vi "BELIKIN FPGA Interface.vi"() -> ()   [LabVIEW 2015]
uses:
  IP Dev Area/IP results.ctl
  <vilib>/Utility/miscctls.llb/LVRectTypeDef.ctl
  <vilib>/userdefined/High Color/IMAQdx.ctl
  <vilib>/FPGAPlugInAG/cRIO-9030/niLvFpga_Open_cRIO-9030.vi
  <vilib>/rvi/interface/common/dynamic/niFpgaDynamicAddResources.vi
  <vilib>/FPGAPlugInAG/Dynamic/niLvFpga_Download_Dynamic.vi
  <vilib>/FPGAPlugInAG/Dynamic/niLvFpga_Run_Dynamic.vi
  <vilib>/Utility/error.llb/Error Cluster From Error Code.vi
  <vilib>/rvi/errors/niLvFpgaAdjustHostInterfaceError.vi
  <vilib>/rvi/interface/nirviOpenFPGA/nirviOpenFPGA.xnode
  FPGA Bitfiles/BELKINEAGLE_FPGATarget_EagleFPGAScanner_Zbij2vyFykg.lvbitx
  <vilib>/rvi/interface/nirviMethod/nirviMethod.xnode
  <vilib>/rvi/interface/nirviReadWriteControl/nirviReadWriteControl.xnode
  <vilib>/rvi/interface/Simulation/niFpgaSimulationCallBeginRW.vi
  NiFpgaLv.dll
panel:
  in  "Scanner Y":dbl(slide)=1.5068493150684925 caption="Y Control" min=-10.0 max=10.0 step=1.0 scale=-10.0..10.0 scale format="%#.3g"
  in  "Scanner X":dbl(slide)=6.712328767123287 caption="X Control" min=-10.0 max=10.0 step=1.0 scale=-10.0..10.0 scale format="%#.3g"
  in  "Red Dots Ctrl":dbl(slide)=1.0 caption="Red Dots" max=10.0 step=1.0 scale=0.01..10.0 scale format="%#.3g"
  in  "V Range Ctrl":dbl(slide)=1.0 caption="V Range" max=10.0 step=1.0 scale=0.01..10.0 scale format="%#.3g"
  in  "LED Ctrl":dbl(slide)=1.0 caption="LED Ring" max=10.0 step=1.0 scale=0.01..10.0 scale format="%#.3g"
  in  "H Range Ctrl":dbl(slide)=1.0 caption="H Range" max=10.0 step=1.0 scale=0.01..10.0 scale format="%#.3g"
  in  "Aiming Ctrl":dbl(slide)=1.0 caption="Aiming" max=10.0 step=1.0 scale=0.01..10.0 scale format="%#.3g"
  out "ViewFinder Sign":picture
  out "Image":T1(plugin-control)
  in  "Center":cluster{"CX":fxp<+,10,10>, "CY":fxp<+,10,10>}
  out "SCAN ENA":bool
  out "X CMD IND":fxp<+/-,20,5>
  out "Y CMD IND":fxp<+/-,20,5>
  out "error out":errorcluster
  in  "Limbus Data":T2={"X"=0, "Y"=0, "A"=100.0, "B"=100.0, "Grade"=0, "Frame#"=0}
  in  "Number Of Points":u16=100
  in  "Fill Elipse":bool
  out "VY CMD":fxp<+/-,32,17>=146.0
  out "VX CMD":fxp<+/-,32,17>=284.0
  out "Stopped":bool=TRUE
  in  "VY OFFS":fxp<+/-,16,1>
  in  "VX OFFS":fxp<+/-,16,1>
  out "Mod3/AI1":fxp<+,18,3>=5.92852783203125
  out "Mod3/AI0":fxp<+,18,3>=3.00372314453125
  out "Y READ":fxp<+/-,20,5>=11.439056396484375
  out "X READ":fxp<+/-,20,5>=14.9774169921875
  in  "Scanner Enable":bool
  in  "Calib Values":T3={"X MULT"=0.008148193359375, "Y MULT"=0.008148193359375, "X OFFS"=0.0, "Y OFFS"=0.0}
  in  "ScanRate":u32=1000
  in  "Y Array":fxp<+/-,10,10>[](array[numeric])=[100.0, 100.0, 99.0, 98.0, 97.0, 95.0, 93.0, 90.0, 88.0, 84.0, 81.0, 77.0, 73.0, 68.0, 64.0, 59.0, 54.0, 48.0, 43.0, 37.0, 31.0, 25.0, 19.0, 13.0, 6.0, 0.0, -6.0, -13.0, -19.0, -25.0, -31.0, -37.0, -43.0, -48.0, -54.0, -59.0, -64.0, -68.0, -73.0, -77.0, -81.0, -84.0, -88.0, -90.0, -93.0, -95.0, -97.0, -98.0, -99.0, -100.0, -100.0, -100.0, -99.0, -98.0, -97.0, -95.0, -93.0, -90.0, -88.0, -84.0, -81.0, -77.0, -73.0, -68.0, -64.0, -59.0, -54.0, -48.0, -43.0, -37.0, -31.0, -25.0, -19.0, -13.0, -6.0, 0.0, 6.0, 13.0, 19.0, 25.0, 31.0, 37.0, 43.0, 48.0, 54.0, 59.0, 64.0, 68.0, 73.0, 77.0, 81.0, 84.0, 88.0, 90.0, 93.0, 95.0, 97.0, 98.0, 99.0, 100.0]
  in  "X Array":fxp<+/-,10,10>[](array[numeric])=[0.0, 6.0, 13.0, 19.0, 25.0, 31.0, 37.0, 43.0, 48.0, 54.0, 59.0, 64.0, 68.0, 73.0, 77.0, 81.0, 84.0, 88.0, 90.0, 93.0, 95.0, 97.0, 98.0, 99.0, 100.0, 100.0, 100.0, 99.0, 98.0, 97.0, 95.0, 93.0, 90.0, 88.0, 84.0, 81.0, 77.0, 73.0, 68.0, 64.0, 59.0, 54.0, 48.0, 43.0, 37.0, 31.0, 25.0, 19.0, 13.0, 6.0, 0.0, -6.0, -13.0, -19.0, -25.0, -31.0, -37.0, -43.0, -48.0, -54.0, -59.0, -64.0, -68.0, -73.0, -77.0, -81.0, -84.0, -88.0, -90.0, -93.0, -95.0, -97.0, -98.0, -99.0, -100.0, -100.0, -100.0, -99.0, -98.0, -97.0, -95.0, -93.0, -90.0, -88.0, -84.0, -81.0, -77.0, -73.0, -68.0, -64.0, -59.0, -54.0, -48.0, -43.0, -37.0, -31.0, -25.0, -19.0, -13.0, -6.0]
  in  "NoGO Zone":T4={"PxMin"=300.0, "PxMax"=300.0, "PyMin"=600.0, "PyMax"=600.0}
  in  "NumOfRetries":u16=5
  in  "stop":bool
  in  "SetSystemValues":bool
  # "EAGLE SYSTEM BASIC CONTROL"
  # "Scanner Control"
  # "Intensity Control"
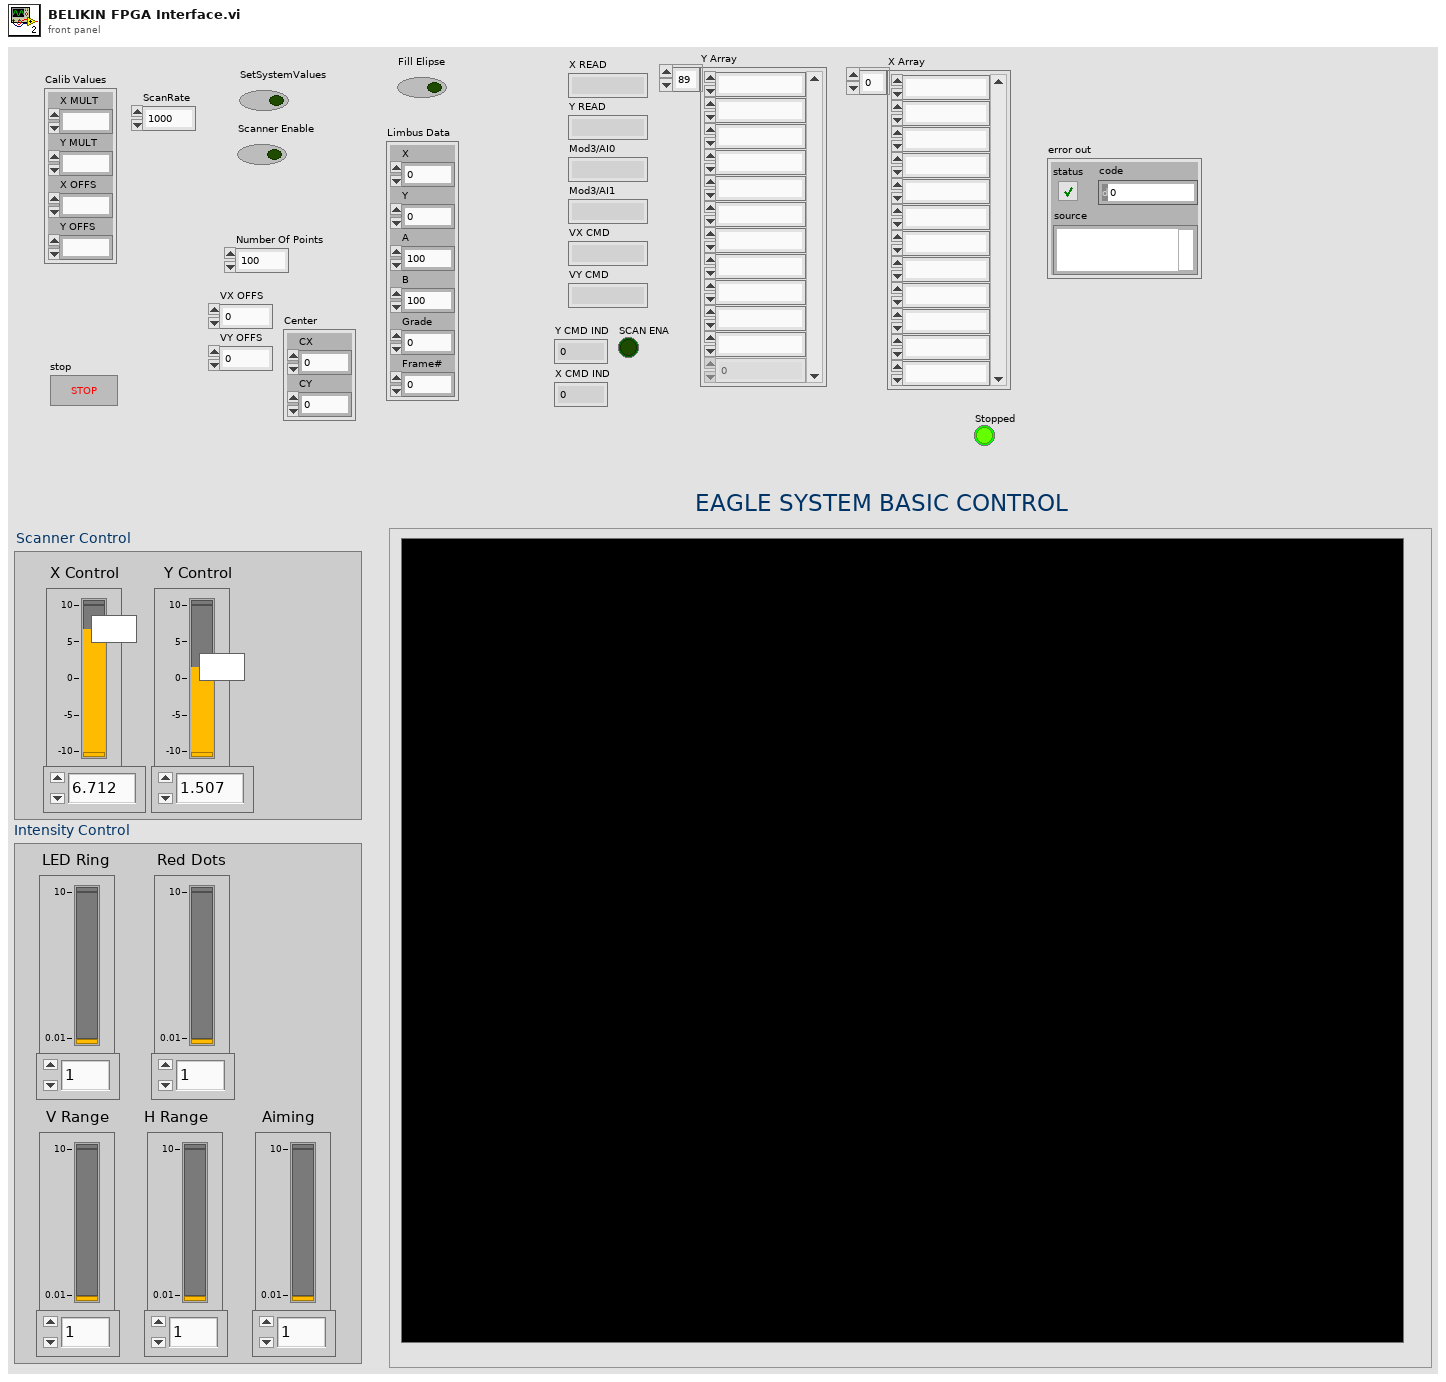
[diagram p1: front panel]
types:
  T1 = typedef "IMAQ Image.ctl" = refnum<image>
  T2 = typedef "IP results.ctl" = cluster{"X":u16, "Y":u16, "A":dbl, "B":dbl, "Grade":u16, "Frame#":u16}
  T3 = cluster{"X MULT":fxp<+/-,20,5>, "Y MULT":fxp<+/-,20,5>, "X OFFS":fxp<+/-,20,5>, "Y OFFS":fxp<+/-,20,5>}
  T4 = cluster{"PxMin":fxp<+,10,10>, "PxMax":fxp<+,10,10>, "PyMin":fxp<+,10,10>, "PyMax":fxp<+,10,10>}
  T5 = typedef "LVRectTypeDef.ctl" = cluster{"Left":i16, "Top":i16, "Right":i16, "Bottom":i16}
  T6 = typedef "IMAQdx.ctl" = refnum<k21>
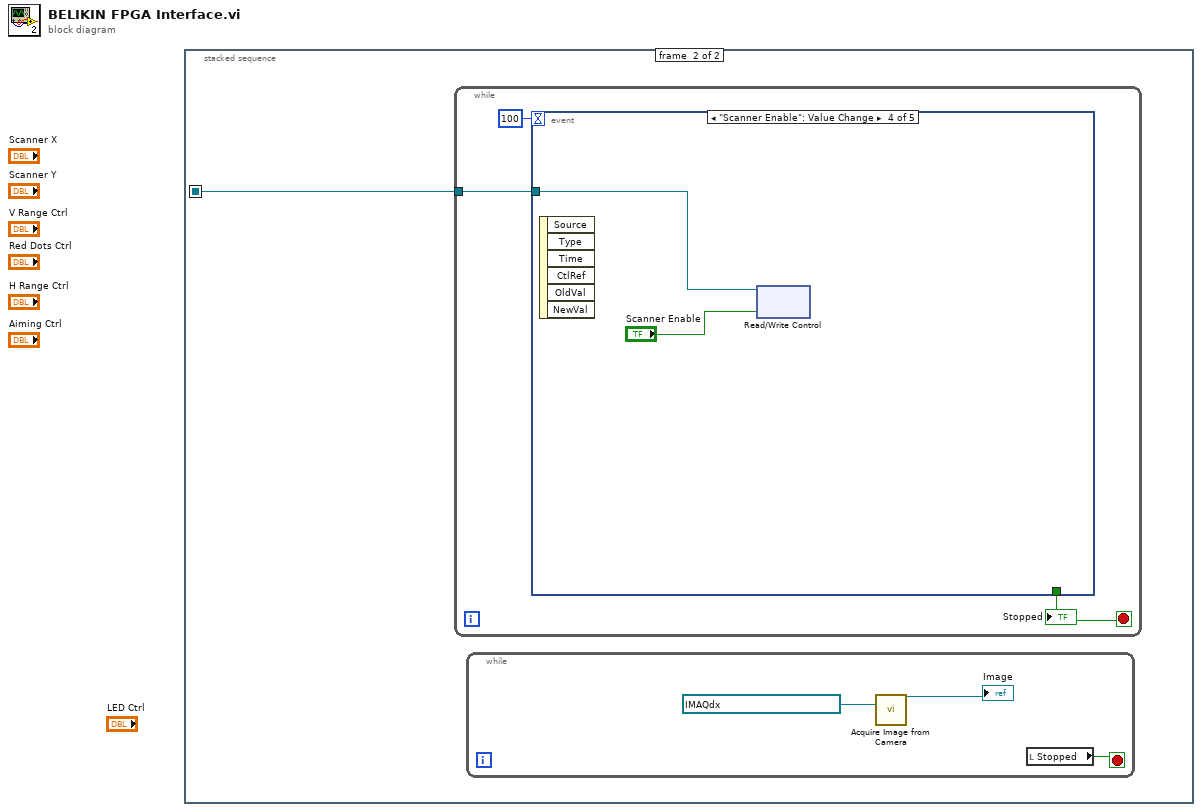
[diagram p0: block diagram]
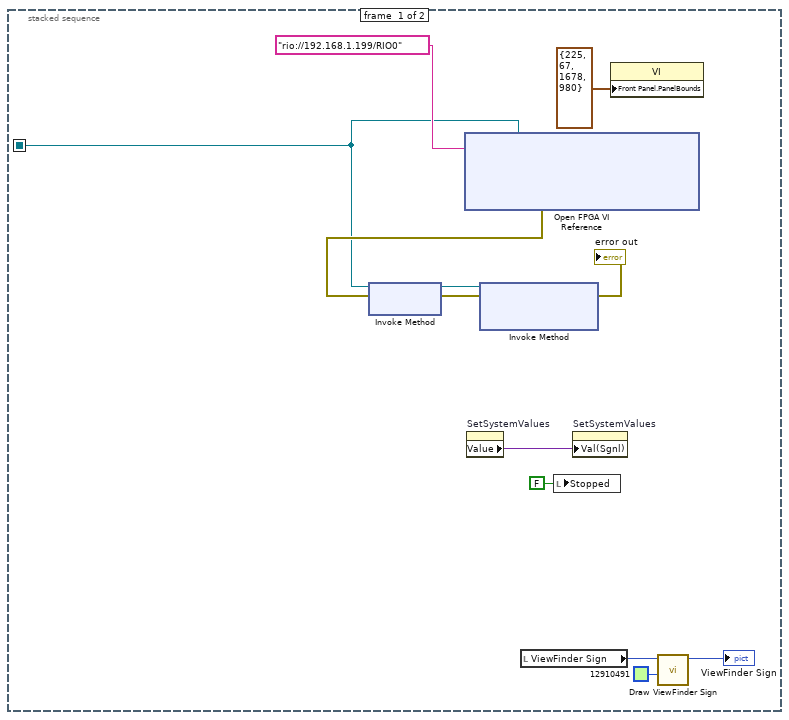
[diagram p2: hidden frame]
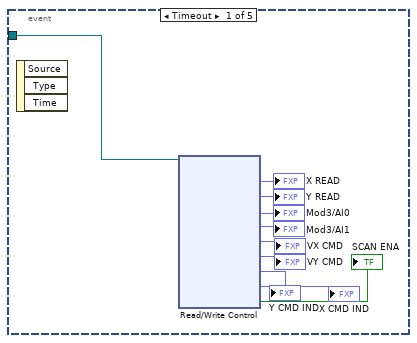
[diagram p3: hidden frame]
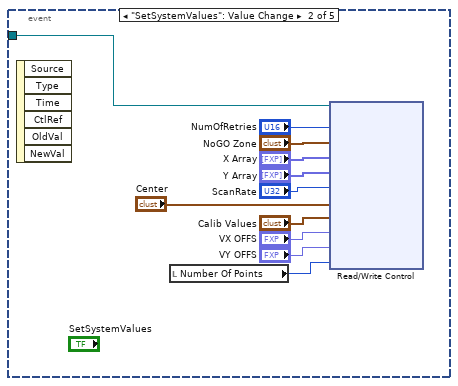
[diagram p4: hidden frame]
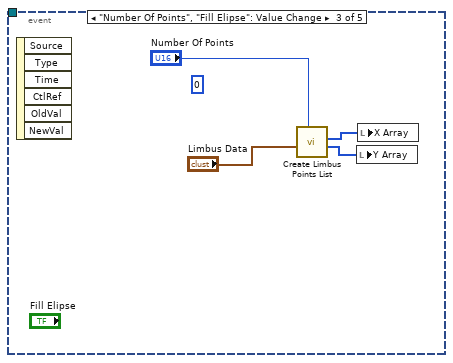
[diagram p5: hidden frame]
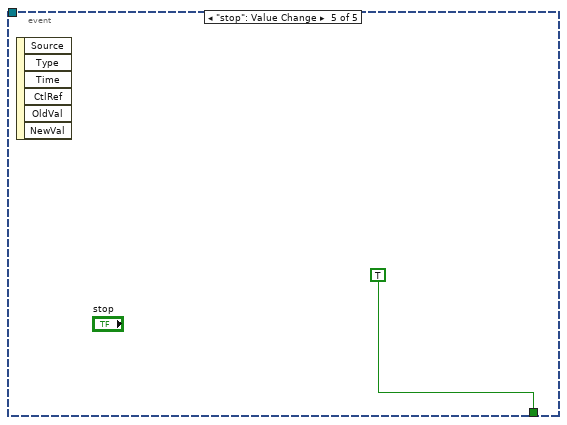
[diagram p6: hidden frame]
diagram:
  n1 = stacked-sequence {
    seq-local: [w5 _] -> [_ w13]
    frame #0 {
      n2 = xnode "Open FPGA VI Reference"("resource name"=tag "rio://192.168.1.199/RIO0") -> ("FPGA VI Reference Out"=w5:refnum<k20>, "error out"=w12:errorcluster)  [unwired: 1 in]
      n3 = xnode "Invoke Method"("FPGA VI Reference In"=w5, "error in"=w12) -> ("FPGA VI Reference Out"=w9:refnum<k20>, "error out"=w11:errorcluster)
      n4 = property on="SetSystemValues" class="Bool"() -> ("Value"=w7:variant)  [unwired: 2 in, 2 out]
      n5 = xnode "Invoke Method"("FPGA VI Reference In"=w9, "error in"=w11) -> ("error out"=→"error out":errorcluster)  [unwired: 1 in, 1 out]
      n6 = local read "ViewFinder Sign"() -> (w1:picture)
      n7 = local write "Stopped"(FALSE ("Stopped")) -> ()
      n8 = property on="SetSystemValues" class="Bool"("Val(Sgnl)"=w7) -> ()  [unwired: 2 in, 2 out]
      n9 = property class="VI"("Front Panel.PanelBounds"=T5 {"Left"=225, "Top"=67, "Right"=1678, "Bottom"=980} ("Front Panel Window:Panel Bounds")) -> ()  [unwired: 2 in, 2 out]
      n10 = call "Draw ViewFinder Sign.vi"("Color"=u32 12910491, "2D Picture"=w1) -> ("2D Picture out"=→"ViewFinder Sign":picture)  [unwired: 9 in]
    }
    frame #1 {
      n11 = while {
        tunnel: w13 -> [w18]
        stop <- w19 stop-if-true
        n12 = event shown="[3] \"Scanner Enable\": Value Change" {
          selector: _ -> [_ _ _ _ _]
          dyn-events: _ -> [_ _ _ _ _]
          timeout: 100 -> [_ _ _ _ _]
          tunnel: [_ _ _ _ TRUE] -> w19
          tunnel: w18 -> [w20 w40 _ w46 _]
          event Timeout {
            n13 = event-data() -> ()  [unwired: 1 in, 3 out]
            n14 = xnode "Read/Write Control"("FPGA VI Reference In"=w20) -> ("X READ"=→"X READ":fxp<+/-,20,5>, "Y READ"=→"Y READ":fxp<+/-,20,5>, "Mod3/AI0"=→"Mod3/AI0":fxp<+,18,3>, "Mod3/AI1"=→"Mod3/AI1":fxp<+,18,3>, "VX CMD"=→"VX CMD":fxp<+/-,32,17>, "VY CMD"=→"VY CMD":fxp<+/-,32,17>, "Y CMD IND"=→"Y CMD IND":fxp<+/-,20,5>, "X CMD IND"=→"X CMD IND":fxp<+/-,20,5>, "SCAN ENA"=→"SCAN ENA":bool)  [unwired: 1 in, 2 out]
          }
          event "SetSystemValues": Value Change {
            n15 = event-data() -> ()  [unwired: 1 in, 6 out]
            n16 = local read "Number Of Points"() -> (w31:u16)
            n17 = xnode "Read/Write Control"("FPGA VI Reference In"=w40, "NumOfRetries"="NumOfRetries", "NoGO Zone"="NoGO Zone", "X Array"="X Array", "Y Array"="Y Array", "ScanRate"="ScanRate", "Center"="Center", "Calib Values"="Calib Values", "VX OFFS"="VX OFFS", "VY OFFS"="VY OFFS", "NoOfPoints"=w31) -> ()  [unwired: 1 in, 2 out]
          }
          event "Number Of Points", "Fill Elipse": Value Change {
            (unwired) u16 0 ("X")
            n18 = event-data() -> ()  [unwired: 1 in, 6 out]
            n19 = call "Create Limbus Points List.vi"("NoOfPoints"="Number Of Points", "IP Results"="Limbus Data") -> ("Y Points"=w42:i16[], "X Points"=w43:i16[])  [unwired: 8 in]
            n20 = local write "Y Array"(w42) -> ()
            n21 = local write "X Array"(w43) -> ()
          }
          event "Scanner Enable": Value Change {
            n22 = event-data() -> ()  [unwired: 1 in, 6 out]
            n23 = xnode "Read/Write Control"("FPGA VI Reference In"=w46, "Reset"="Scanner Enable") -> ()  [unwired: 1 in, 2 out]
          }
          event "stop": Value Change {
            n24 = event-data() -> ()  [unwired: 1 in, 6 out]
          }
        }
        "Stopped" <- w19
      }
      n25 = while {
        stop <- w14 stop-if-true
        n26 = call "Acquire Image from Camera.vi"("Session In"=T6 "rio:\\\\192.168.1.199\\cam0") -> ("Image Out"=→"Image":T1)  [unwired: 23 in, 3 out]
        n27 = local read "Stopped"() -> (w14:bool)
      }
    }
  }
